vi "dll.midi_get_input_device_count.vi"(8 "error in (no error)":errorcluster, 11 "LabVIEW-MIDI-XPLAT in":refnum<class "midi in.lvclass">) -> (0 "error out":errorcluster, 2 "device count":i32, 3 "LabVIEW-MIDI-XPLAT out":refnum<class "midi in.lvclass">)   [LabVIEW 2020, in "midi in.lvclass"]
uses:
  midi in.lvclass
  midi in.lvclass/midi in.ctl
  shared/midi shared.lvlib
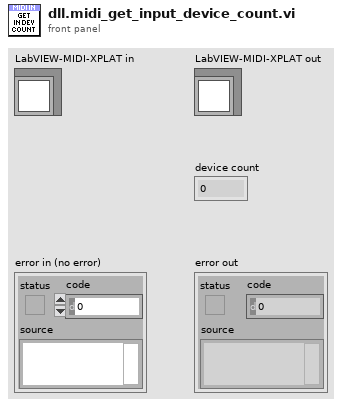
[diagram p1: front panel]
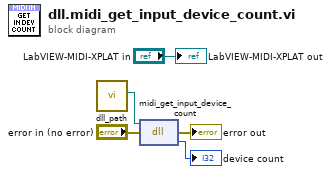
[diagram p0: block diagram]
diagram:
  n1 = call "dll_path.vi"() -> ("dll"=w1:path)  [unwired: 11 in]
  n2 = dll-call lib="C:/code/LabVIEW-MIDI-XPLAT/dist/TomMIDIllan_*.*" fn="midi_get_input_device_count"(path in=w1, error in="error in (no error)") -> (error out=→"error out":errorcluster, "device count"=→"device count":i32)  [unwired: 1 in, 1 out]
  "LabVIEW-MIDI-XPLAT out" <- "LabVIEW-MIDI-XPLAT in"
